vi "ExposeMapperGetDefaultValue.vi"(11 "Data Val Ref in":refnum<data-value>) -> (3 "Data Val Ref Out":refnum<data-value>)   [LabVIEW 2017]
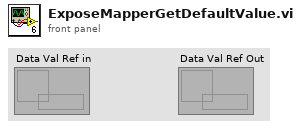
[diagram p1: front panel]
types:
  T1 = typedef "ExposeMapperDataTypeEnum.ctl" = enum16{"NotData", "int8", "byte", "int16", "uint16", "int32", "uint32", "int64", "uint64", "Single", "Double", "String", "Boolean", "Container"}
  T2 = typedef "ExposeObjectMapContainerTypeEnum.ctl" = enum16{"Value", "Array", "Waveform", "NetContainer"}
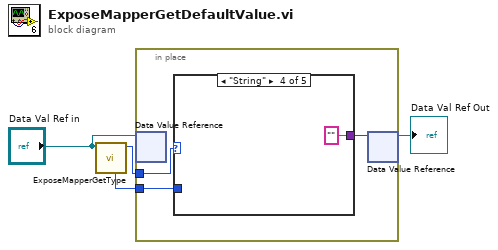
[diagram p0: block diagram]
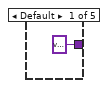
[diagram p2: hidden frame]
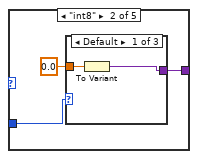
[diagram p3: hidden frame]
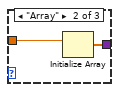
[diagram p4: hidden frame]
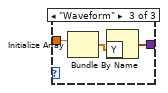
[diagram p5: hidden frame]
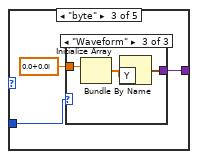
[diagram p6: hidden frame]
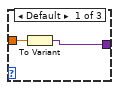
[diagram p7: hidden frame]
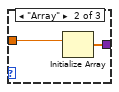
[diagram p8: hidden frame]
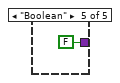
[diagram p9: hidden frame]
diagram:
  n1 = call "ExposeMapperGetType.vi"("Data Val Ref in"="Data Val Ref in") -> ("DataType"=w3:T1, "Container Type (Labview Value type)"=w2:T2)  [unwired: 5 in, 4 out]
  n2 = in-place {
    in-place-border: w3 -> [w6]
    in-place-border: w2 -> [w5]
    n3 = in-place-dvr #1("Data Val Ref in") -> ()  [unwired: 2 out]
    n4 = case shown="\"String\"" w6 {
      tunnel: [variant w9 w19 "" FALSE] -> w7
      tunnel: w5 -> [_ w11 w21 _ _]
      frame Default {
      }
      frame "int8" {
        n5 = case shown="Default" w11 {
          tunnel: 0.0 -> [w13 w15 w18]
          tunnel: [w12 w14 w16] -> w9
          frame Default {
            n6 = To Variant(anything=w13) -> (Variant=w12:variant)
          }
          frame "Array" {
            n7 = Initialize Array(w15) -> (w14:dbl[])  [unwired: 1 in]
          }
          frame "Waveform" {
            n8 = Initialize Array(w18) -> (w17:dbl[])  [unwired: 1 in]
            n9 = Bundle By Name("Y"=w17) -> (w16:waveform(dbl))  [unwired: 1 in]
          }
        }
      }
      frame "byte" {
        n10 = case shown="\"Waveform\"" w21 {
          tunnel: cdb 0.0+0.0i -> [w23 w25 w28]
          tunnel: [w22 w24 w26] -> w19
          frame Default {
            n11 = To Variant(anything=w23) -> (Variant=w22:variant)
          }
          frame "Array" {
            n12 = Initialize Array(w25) -> (w24:cdb[])  [unwired: 1 in]
          }
          frame "Waveform" {
            n13 = Initialize Array(w28) -> (w27:cdb[])  [unwired: 1 in]
            n14 = Bundle By Name("Y"=w27) -> (w26:waveform(cdb))  [unwired: 1 in]
          }
        }
      }
      frame "String" {
      }
      frame "Boolean" {
      }
    }
    n15 = in-place-dvr #1(w7) -> (→"Data Val Ref Out":refnum<data-value>)  [unwired: 1 out]
  }
